vi "Spectrograph_getEvent_detailedState.vi"(8 "error in (no error)":errorcluster, 11 "logevent_detailedState_Ctl":T1) -> (0 "error out":errorcluster, 2 "function return":i32, 3 "logevent_detailedState_Ctl out":T1)   [LabVIEW 2016, in "SALLV_Spectrograph.lvlib"]
doc: "int Spectrograph_shm_getEvent_detailedStateLV(Spectrograph_logevent_detailedStateLV *logevent_detailedState_Ctl );"
uses:
  SALLV_Spectrograph.lvlib
  DataTypes/logevent_detailedState.ctl
  SALLV_Spectrograph.so
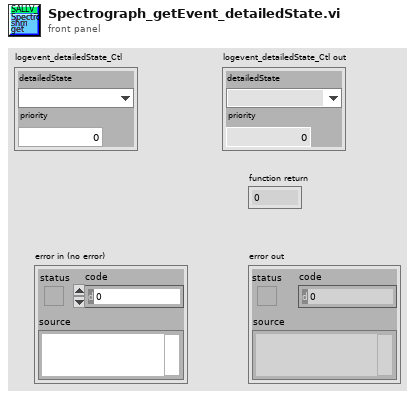
[diagram p1: front panel]
types:
  T1 = typedef "SALLV_Spectrograph.lvlib/logevent_detailedState.ctl" = cluster{"detailedState":enum32{"", "DisabledState", "EnabledState", "FaultState", "OfflineState", "StandbyState", "stationaryState", "movingState"}, "priority":i32}
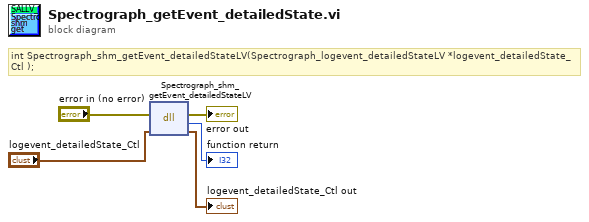
[diagram p0: block diagram]
diagram:
  # "int Spectrograph_shm_getEvent_detailedStateLV(Spectrograph_logevent_detailedStateLV *logevent_detailedState_Ctl );"
  n1 = dll-call lib="home/harini/TCS/SALLV_Spectrograph/SALLV_Spectrograph.*" fn="Spectrograph_shm_getEvent_detailedStateLV"(error in="error in (no error)", "logevent_detailedState_Ctl"="logevent_detailedState_Ctl") -> (error out=→"error out":errorcluster, →"function return":i32, "logevent_detailedState_Ctl"=→"logevent_detailedState_Ctl out":T1)  [unwired: 2 in, 1 out]
